vi "Write SubSampling Interval.vi"(8 "error in (no error)":errorcluster, 10 "SubSampling Interval":i32, 11 "Roughness Averager in":refnum<class "Roughness Averager.lvclass">) -> (0 "error out":errorcluster, 3 "Roughness Averager out":refnum<class "Roughness Averager.lvclass">)   [LabVIEW 2018, in "Roughness Averager.lvclass"]
uses:
  Roughness Averager.lvclass
  Roughness Averager.lvclass/Roughness Averager.ctl
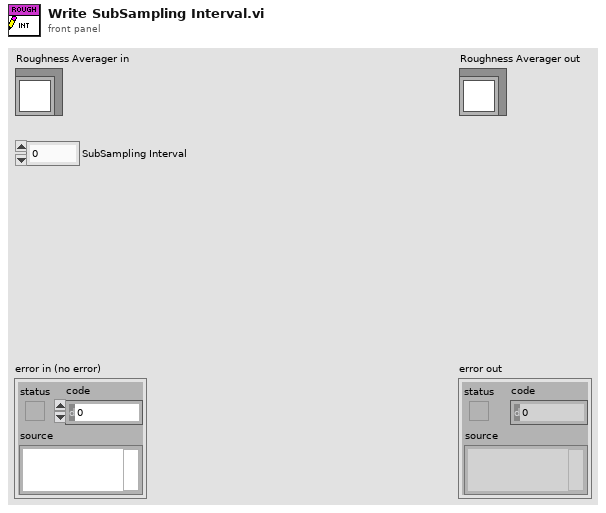
[diagram p1: front panel]
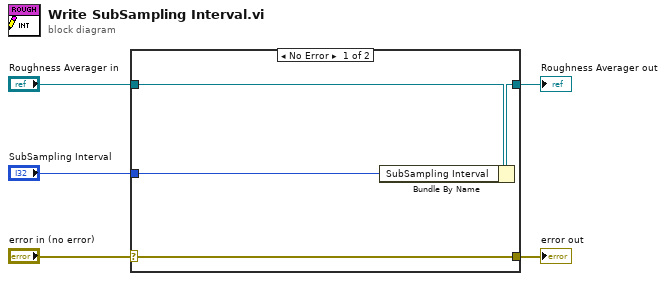
[diagram p0: block diagram]
diagram:
  n1 = case shown="No Error" "error in (no error)" {
    selector: "error in (no error)" -> [w9 w10]
    tunnel: [w9 w10] -> w4
    tunnel: [w7 w11] -> w2
    tunnel: "Roughness Averager in" -> [w8 w11]
    tunnel: "SubSampling Interval" -> [w6 _]
    frame No Error {
      n2 = Bundle By Name(cluster=w8, "SubSampling Interval"=w6) -> (w7:refnum<class "Roughness Averager.lvclass">)
    }
    frame Error {
    }
  }
  "error out" <- w4
  "Roughness Averager out" <- w2
